vi "AppState.vi"() -> ()   [LabVIEW 2012]
panel:
  in  "AppState":u16
  # "Idle: 0\nCalibration, idle: 1\nMesure: 2\nCalibration, mesure: 4\nExport: 5"
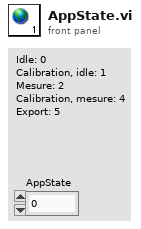
[diagram p1: front panel]
diagram:
